vi "Get Attribute VAR.vi"(8 "error in":errorcluster, 9 "Data Type and Default Value":variant, 10 "Attribute":string, 11 "Config from EXCEL in":refnum<class "Config from EXCEL.lvclass">) -> (0 "error out":errorcluster, 2 "Value":variant, 3 "Config from EXCEL out":refnum<class "Config from EXCEL.lvclass">)   [LabVIEW 2019, in "Config from EXCEL.lvclass"]
uses:
  Config from EXCEL.lvclass
  Config from EXCEL.lvclass/Config from EXCEL.ctl
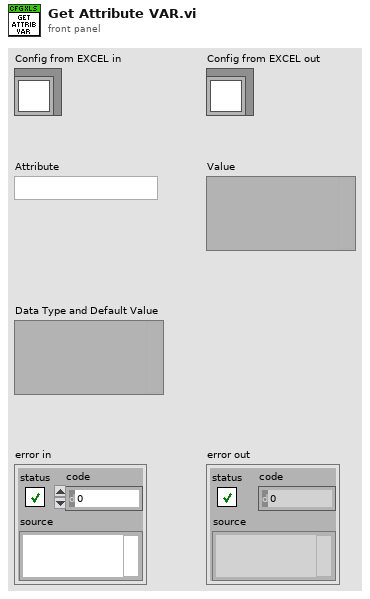
[diagram p1: front panel]
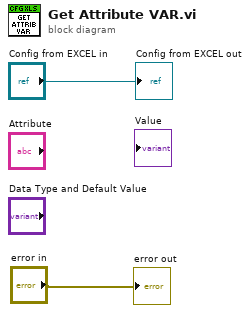
[diagram p0: block diagram]
diagram:
  "error out" <- "error in"
  "Config from EXCEL out" <- "Config from EXCEL in"
